vi "sub_int32.vi"() -> ()   [LabVIEW 2019]
uses:
  <vilib>/RTI DDS Toolkit/Types/RTI DDS Advanced Reader Configuration.ctl
  <vilib>/RTI DDS Toolkit/Types/DDS Sample Info.ctl
  <vilib>/RTI DDS Toolkit/VIs/AdvancedCreateReader_NumI32.vi
  <vilib>/RTI DDS Toolkit/VIs/Read_NumI32.vi
  <vilib>/RTI DDS Toolkit/Library/LVDDS_library.lvlib
panel:
  out "n":i32
  out "DDS Sample Info":T1={"DDS_SampleStateKind"=enum."DDS_READ_SAMPLE_STATE", "DDS_ViewStateKind"=enum."DDS_NOT_NEW_VIEW_STATE", "DDS_InstanceStateKind"=enum."DDS_ALIVE_INSTANCE_STATE", "sec"=1655201026, "nanosec"=165925821, "valid_data"=TRUE}
  out "Data":i32=557
  in  "stop":bool
  in  "dt":u32=100
  in  "Topic Name":string="rt/rosint32"
  in  "config":T2={"typeName"="std_msgs::msg::dds_::Int32_", "keyName"="", "domainParticipantQoSProfile"="", "dataReaderQoSProfile"="", "forceArrayMapping?"=FALSE, "forceExclusiveReader?"=FALSE, "forceRead? (only ExclusiveReader)"=FALSE, "forceUnboundedString?"=FALSE}
  # "Source Timestamp"
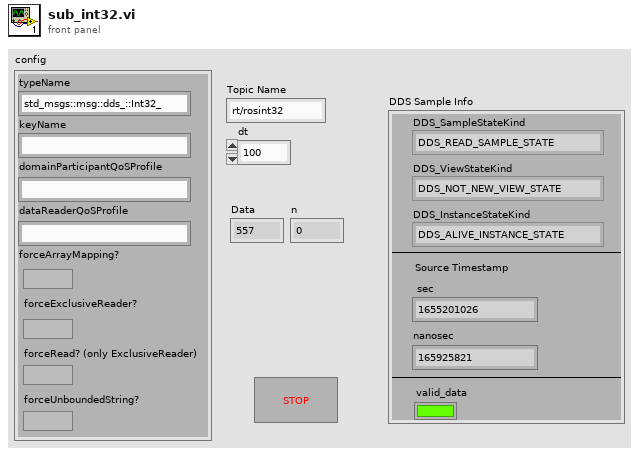
[diagram p1: front panel]
types:
  T1 = typedef "LVDDS_library.lvlib/DDS Sample Info.ctl" = cluster{"DDS_SampleStateKind":enum32{"DDS_INVALID_SAMPLE_STATE", "DDS_READ_SAMPLE_STATE", "DDS_NOT_READ_SAMPLE_STATE"}, "DDS_ViewStateKind":enum32{"DDS_INVALID_SAMPLE_STATE", "DDS_NEW_VIEW_STATE", "DDS_NOT_NEW_VIEW_STATE"}, "DDS_InstanceStateKind":enum32{"DDS_INVALID_STATE", "DDS_ALIVE_INSTANCE_STATE", "DDS_NOT_ALIVE_DISPOSED_INSTANCE_STATE", "", "DDS_NOT_ALIVE_NO_WRITERS_INSTANCE_STATE"}, "sec":i32, "nanosec":u32, "valid_data":bool}
  T2 = typedef "LVDDS_library.lvlib/RTI DDS Advanced Reader Configuration.ctl" = cluster{"typeName":string, "keyName":string, "domainParticipantQoSProfile":string, "dataReaderQoSProfile":string, "forceArrayMapping?":bool, "forceExclusiveReader?":bool, "forceRead? (only ExclusiveReader)":bool, "forceUnboundedString?":bool}
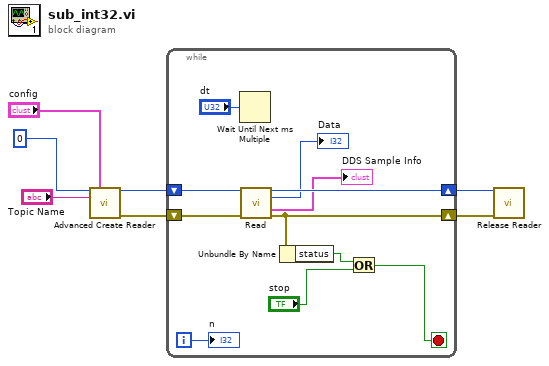
[diagram p0: block diagram]
diagram:
  n1 = call-poly <vilib>:"Advanced Create Reader.vi"("Domain Id"=u32 0, "Advanced Reader Configuration"="config", "Topic Name"="Topic Name") -> ("DDS Object Ref"=w7:u64, "error out"=w4:errorcluster)  [unwired: 11 in]
  n2 = while {
    shift-right: [w17] -> w6
    shift-left: w7 -> [w18]
    shift-right: [w14] -> w5
    shift-left: w4 -> [w16]
    i -> [w8]
    stop <- w12 stop-if-true
    n3 = Wait Until Next ms Multiple(millisecond multiple="dt") -> ()  [unwired: 1 out]
    n4 = call-poly <vilib>:"Read.vi"("DDS Object Ref in"=w18, "error in (no error)"=w16) -> ("DDS Object Ref out"=w17:u64, "Data"=→"Data":i32, "DDS Sample Info"=→"DDS Sample Info":T1, "error out"=w14:errorcluster)  [unwired: 9 in, 1 out]
    n5 = Unbundle By Name(w14) -> ("status"=w13:bool)
    n6 = Or(x=w13, y="stop") -> (x .or. y?=w12:bool)
    "n" <- w8
  }
  n7 = call <vilib>:"Release Reader.vi"("error in (no error)"=w5, "DDS Object Ref"=w6) -> ()  [unwired: 9 in, 1 out]
